vi "handshake_final.vi"(6 "protocol_version":i32, 8 "error in (no error)":errorcluster, 9 "client_first_message":string, 10 "password":string, 11 "server_response (json)":string="{\"success\":true,\"min_protocol_version\":0,\"max_protocol_version\":0,\"server_version\":\"2.3.0\"}\u0000\n{\"success\":true,\"authentication\":\"r=rOprNGfwEbeRWgbNEkqO%hvYDpWUa2RaTCAfuxFIlj)hNlF$k0,s=W22ZaJ0SNY7soEsUEjb6gQ==,i=4096\"}\u0000") -> (0 "error out":errorcluster, 3 "authentication_request":string)   [LabVIEW 2017, in "rethinkdb.lvlib"]
uses:
  rethinkdb.lvlib
  9ccb81d9-1f4e-42d0-81b4-a094be45088c.vi
  e7072015-6297-4b13-a5d2-66322d8040fe.vi
  817db7f3-f43c-4758-8d67-4fcbd3026d38.vi
  json_get_names.vi
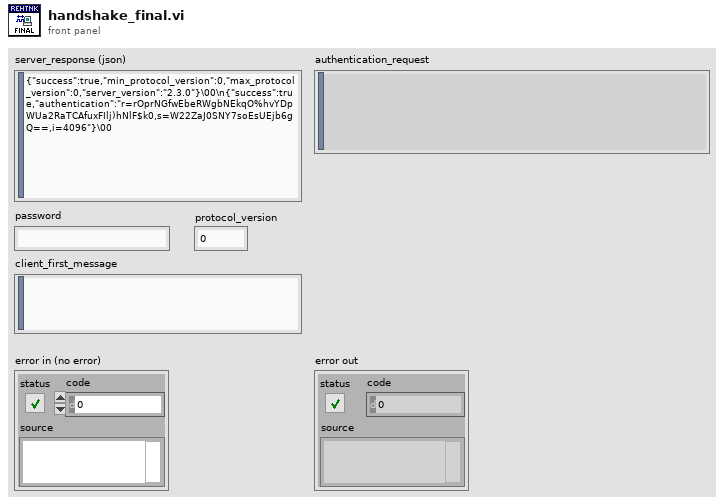
[diagram p1: front panel]
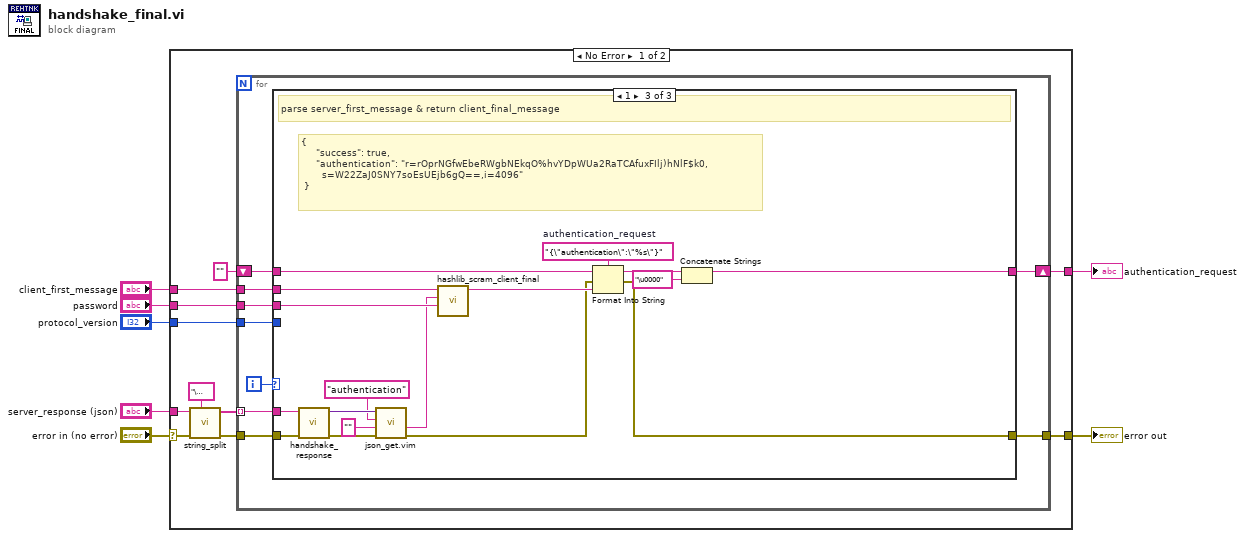
[diagram p0: block diagram]
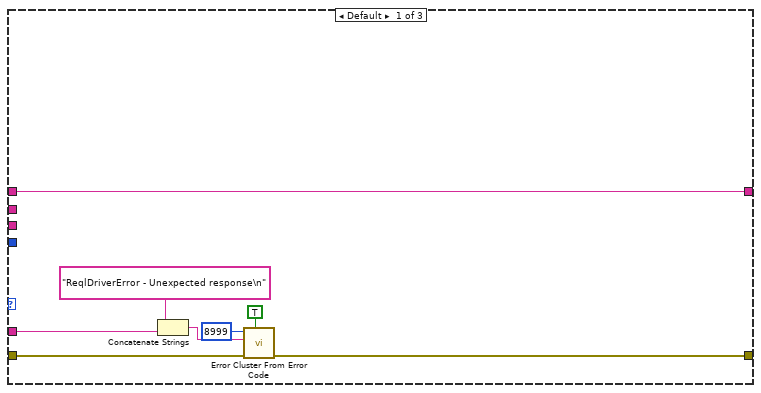
[diagram p2: hidden frame]
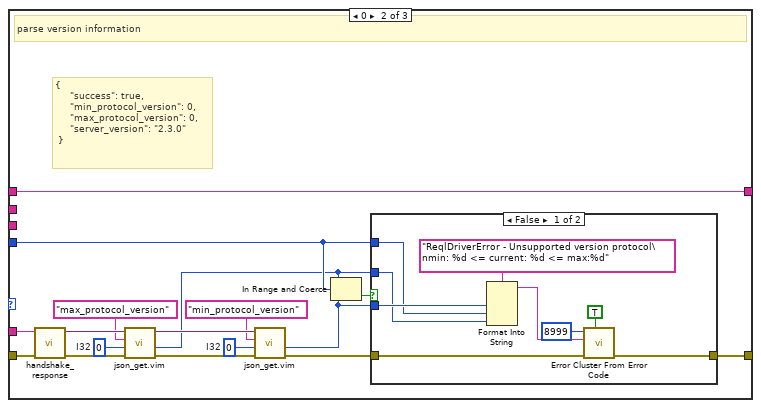
[diagram p3: hidden frame]
diagram:
  n1 = case shown="No Error" "error in (no error)" {
    selector: "error in (no error)" -> [w9 w79]
    tunnel: [w16 w79] -> w6
    tunnel: [w15 _] -> w5
    tunnel: "server_response (json)" -> [w17 _]
    tunnel: "client_first_message" -> [w13 _]
    tunnel: "password" -> [w12 _]
    tunnel: "protocol_version" -> [w10 _]
    frame No Error {
      n2 = call "string_split.vi"("char (0x00)"="\u0000", "data in"=w17) -> ("messages"=w14:string[])  [unwired: 8 in, 1 out]
      n3 = for {
        tunnel: [w26] -> w16
        tunnel: w14 -> [w21] mode=indexing
        tunnel: w12 -> [w23]
        tunnel: w9 -> [w22]
        tunnel: w13 -> [w24]
        shift-right: [w25] -> w15
        shift-left: "" -> [w19]
        tunnel: w10 -> [w18]
        i -> [w20]
        n4 = case shown="1" w20 {
          tunnel: [w28 w48 w78] -> w26
          tunnel: [w27 w49 w77] -> w25
          tunnel: w24 -> [_ _ w72]
          tunnel: w23 -> [_ _ w71]
          tunnel: w22 -> [w30 w51 w70]
          tunnel: w21 -> [w29 w50 w69]
          tunnel: w19 -> [w27 w49 w68]
          tunnel: w18 -> [_ w46 _]
          frame Default {
            n5 = Concatenate Strings("ReqlDriverError - Unexpected response\n" ("error message (\"\")"), w29) -> (w31:string)
            n6 = call <vilib>:"Error Cluster From Error Code.vi"("show call chain? (False)"=TRUE, "error in (no error)"=w30, "error message (\"\")"=w31, "error code (0)"=8999) -> ("error out"=w28:errorcluster)  [unwired: 5 in]
          }
          frame 0 {
            w39 = 0  # I32
            w43 = 0  # I32
            # "{\n     \"success\": true,\n     \"min_protocol_version\": 0,\n     \"max_protocol_version\": 0,\n     \"server_version\": \"2.3.0\"\n }"
            # "parse version information"
            n7 = call "handshake_response.vi"("error in (no error)"=w51, "response"=w50) -> ("error out"=w45:errorcluster, "value"=w44:variant)  [unwired: 8 in]
            n8 = call "json_get.vim"("error in (no error)"=w45, "default"=w43, "name"="max_protocol_version" ("key"), "variant in"=w44) -> ("error out"=w41:errorcluster, "value"=w36:i32, "variant out"=w38:variant)  [unwired: 4 in, 1 out]
            n9 = call "json_get.vim"("error in (no error)"=w41, "default"=w39, "name"="min_protocol_version" ("key"), "variant in"=w38) -> ("error out"=w40:errorcluster, "value"=w35:i32)  [unwired: 4 in, 2 out]
            n10 = In Range and Coerce(upper limit=w36, x=w46, lower limit=w35) -> (In Range?=w47:bool)  [unwired: 1 out]
            n11 = case shown="False" w47 {
              tunnel: [w57 w61] -> w48
              tunnel: w40 -> [w58 w61]
              tunnel: w35 -> [w56 _]
              tunnel: w46 -> [w53 _]
              tunnel: w36 -> [w52 _]
              frame False {
                n12 = Format Into String(format string="ReqlDriverError - Unsupported version protocol\nmin: %d <= current: %d <= max:%d" ("error message (\"\")"), w56, w53, w52) -> (resulting string=w54:string)  [unwired: 2 in, 1 out]
                n13 = call <vilib>:"Error Cluster From Error Code.vi"("show call chain? (False)"=TRUE, "error in (no error)"=w58, "error message (\"\")"=w54, "error code (0)"=8999) -> ("error out"=w57:errorcluster)  [unwired: 5 in]
              }
              frame True {
                # "supported protocol version"
              }
            }
          }
          frame 1 {
            w76 = "{\"authentication\":\"%s\"}"  # authentication_request
            # "{\n     \"success\": true,\n     \"authentication\": \"r=rOprNGfwEbeRWgbNEkqO%hvYDpWUa2RaTCAfuxFIlj)hNlF$k0,\n       s=W22ZaJ0SNY7soEsUEjb6gQ==,i=4096\"\n }"
            # "parse server_first_message & return client_final_message"
            n14 = call "handshake_response.vi"("error in (no error)"=w70, "response"=w69) -> ("error out"=w67:errorcluster, "value"=w66:variant)  [unwired: 8 in]
            n15 = call "json_get.vim"("error in (no error)"=w67, "default"="", "name"="authentication" ("key"), "variant in"=w66) -> ("error out"=w64:errorcluster, "value"=w63:string)  [unwired: 4 in, 2 out]
            n16 = call "hashlib_scram_client_final.vi"("password"=w71, "server_first_message"=w63, "client_first_message"=w72) -> ("client_final_message"=w73:string)  [unwired: 8 in]
            n17 = Format Into String(format string=w76, initial string=w68, error in=w64, w73) -> (resulting string=w75:string, error out=w78:errorcluster)
            n18 = Concatenate Strings(w75, "\u0000" ("string")) -> (w77:string)
          }
        }
      }
    }
    frame Error {
    }
  }
  "error out" <- w6
  "authentication_request" <- w5
